vi "Set Correct IPG Temp Cals.vi"(6 "Gen Cals In":string="Reserved[00]=0x00\nReserved[01]=0x00\nReserved[02]=0x00\nReserved[03]=0x00\nReserved[04]=0x00\nReserved[05]=0x00\nReserved[06]=0x00\nReserved[07]=0x00\nReserved[08]=0x00\t\t\nReserved[09]=0x00\nReserved[10]=0x00\nReserved[11]=0x00\nReserved[12]=0x00\nReserved[13]=0x00\nReserved[14]=0x00\ntempMinThreshold=0xCAC4\ntempWarningThresholdl=0x31D3\ntempCriticalThresholdl=0x2FBB\ntempAbortThresholdl=0x2DBD\nthermOffsetMinimum=0x190\nthermOffsetMaximum=0x320\nthermBiasMinimum=0x3E8\nthermBiasMaximum=0xD48\nthermInputMinimum=0x384\nthermInputMaximum=0xC1C\nbatteryIncreasePreCharge=0x19\nbatteryIncreaseConstandCurrent=0x08\nReserved[00]=0x00\nReserved[01]=0x00\nReserved[02]=0x00\nReserved[03]=0x00\nReserved[04]=0x00\nReserved[05]=0x00\nReserved[06]=0x00\nReserved[07]=0x00\nReserved[08]=0x00\nReserved[09]=0x00\nReserved[10]=0x00\nReserved[11]=0x00\nReserved[12]=0x00\nReserved[13]=0x00\nReserved[14]=0x00\nbatteryStateCalStimOff[00]=0xCDE\nbatteryStateCalStimOff[01]=0xC8B\nbatteryStateCalStimOff[02]=0xC4F\nbatteryStateCalStimOff[03]=0xC2E\nbatteryStateCalStimOff[04]=0xC0C\nbatteryStateCalStimOff[05]=0x948\nbatteryStateCalStimOn[00]=0xCCB\nbatteryStateCalStimOn[01]=0xC75\nbatteryStateCalStimOn[02]=0xC3B\nbatteryStateCalStimOn[03]=0xC19\nbatteryStateCalStimOn[04]=0xBFC\nbatteryStateCalStimOn[05]=0x948\nvrectMeasurementCal=0x2EE", 7 "Cal Minimum Threshold (R/4)":string="NaN", 8 "error in":errorcluster, 9 "Cal Abort Threshold (R/4)":string="NaN", 10 "Cal Critical Threshold (R/4)":string="NaN", 11 "Cal Warning Threshold (R/4)":string="NaN") -> (0 "error out":errorcluster)   [LabVIEW 2010]
uses:
  Drivers/Telemetry/Typedef Command List.ctl
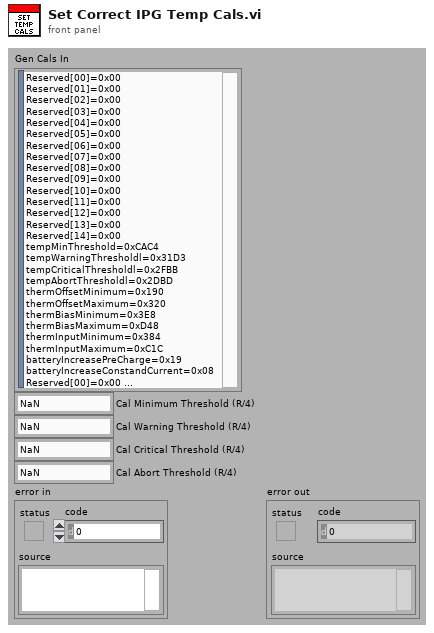
[diagram p1: front panel]
types:
  T1 = typedef "Typedef Command List.ctl" = enum16{"Get xPG Status", "xPG Stimulation", "Select Program", "Increment Program Amplitude", "Decrement Program Amplitude", "Get PoP Constants", "Get PPC Constants", "Get Program Names", "Set Pulse Amplitude", "Increment Pulse Amplitude", "Decrement Pulse Amplitude", "Get Pulse Widths", "Set Pulse Widths", "Increment Pulse Width", "Decrement Pulse Width", "Get Program Frequency", "Set Program Frequency", "Increment Program Frequency", "Decrement Program Frequency", "Inject Event", "Charging Control", "Get xPG Identity", "Set xPG Identity", "Restore Program Defaults", "Get Program Definition", "Set Program Definition", "Get Program Constants", "Set Program Constants", "Get Configurable Device Parameters", "Set Configurable Device Parameters", "Get Pulse Constants", "Set Pulse Constants", "Get Lead Limits", "Set Lead Limits", "Get Channel Calibrations", "Set Channel Calibrations", "<reserved 2>", "<reserved 3>", "<reserved 4>", "<reserved 5>", "<reserved 6>", "<reserved 7>", "Get Stim Asic HV Calibrations", "Set Stim Asic HV Calibrations", "<reserved 8>", "<reserved 9>", "Get CP Data", "Set CP Data", "Clear Log", "Read Log", "Append Log", "Get Patient Program Runtime", "Set Patient Program Runtime", "Impedance Measurement", "Enter Storage Mode", "Echo Short", "Echo Long", "Get General Calibration", "Set General Calibration", "Get Trim List", "Set Trim List", "Get Counter", "Set Counter", "Get Test Stimulation", "Set Test Stimulation", "Get Titration Stimulation", "Set Titration Stimulation", "Get Ramp Time", "Set Ramp Time", "Get VBAT", "Set Software Description Block", "Get Software Description Block", "Write Memory", "Read Memory", "Reset xPG", "Erase Flash Block", "Write Vectors", "Read Vectors", "Diagnostic Data", "Set Background Impedance", "Get Background Impedence ", "Set Test Waveform", "Calibrate Channel", "Get Log Range", "Reserved 0x55", "Reserved 0x56", "MICS Options", "Pair PPC", "Pair POP", "Stop Bootloader", "Tune MICS", "MICS Diagnostics", "Undefined"}
  T2 = cluster{"Command":T1, "Function":enum16{"Open Session", "Close Session", "Downlink Only", "Uplink Only", "Transceive (DN -> UP)"}, "MICS_ID":u32, "EXID":u32, "Use Local":bool, "Transceive Delay mS":dbl, "CP_DATA IN":u8[], "Parameters":string}
  T3 = enum16{"Open Session", "Close Session", "Downlink Only", "Uplink Only", "Transceive (DN -> UP)"}
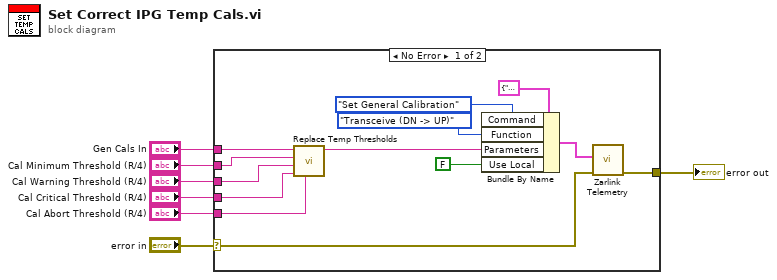
[diagram p0: block diagram]
diagram:
  n1 = case shown="No Error" "error in" {
    selector: "error in" -> [w9 w21]
    tunnel: "Gen Cals In" -> [w14 _]
    tunnel: "Cal Minimum Threshold (R/4)" -> [w13 _]
    tunnel: "Cal Warning Threshold (R/4)" -> [w12 _]
    tunnel: "Cal Critical Threshold (R/4)" -> [w11 _]
    tunnel: "Cal Abort Threshold (R/4)" -> [w10 _]
    tunnel: [w8 w21] -> w1
    frame No Error {
      n2 = call "Replace Temp Thresholds.vi"("Cal Abort Threshold (R/4)"=w10, "Cal Critical Threshold (R/4)"=w11, "Cal Warning Threshold (R/4)"=w12, "Cal Minimum Threshold (R/4)"=w13, "Gen Cals In"=w14) -> ("Gen Cals Out"=w15:string)  [unwired: 6 in]
      n3 = Bundle By Name(cluster=T2 {"Command"=enum."Get xPG Status", "Function"=enum."Close Session", "MICS_ID"=0, "EXID"=16773121, "Use Local"=FALSE, "Transceive Delay mS"=100.0, "CP_DATA IN"=[], "Parameters"=""} ("Input"), "Command"=Typedef_Command_List."Set General Calibration", "Function"=T3."Transceive (DN -> UP)", "Parameters"=w15, "Use Local"=FALSE) -> (w20:T2)
      n4 = call "Zarlink Telemetry.vi"("error in (no error)"=w9, "Input"=w20) -> ("error out"=w8:errorcluster)  [unwired: 7 in, 2 out]
    }
    frame Error {
    }
  }
  "error out" <- w1
